vi "TestTCP.vi"() -> ()   [LabVIEW 2020]
panel:
  out "error out":errorcluster
  out "data out1":string
  out "loop2":i32
  out "loop1":i32
  out "data out 2":string
  in  "Stop loop 2":bool
  in  "Stop loop1":bool
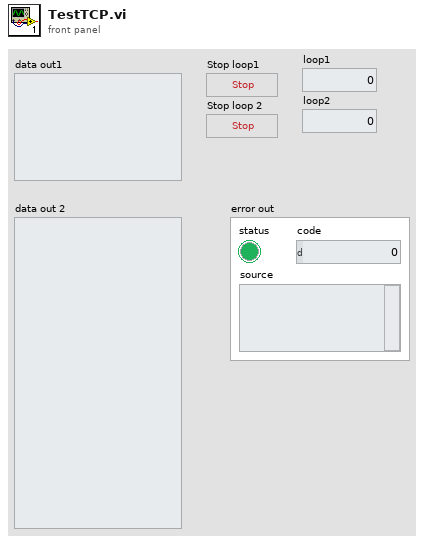
[diagram p1: front panel]
types:
  T1 = enum16{"Standard", "Buffered", "CRLF", "Immediate"}
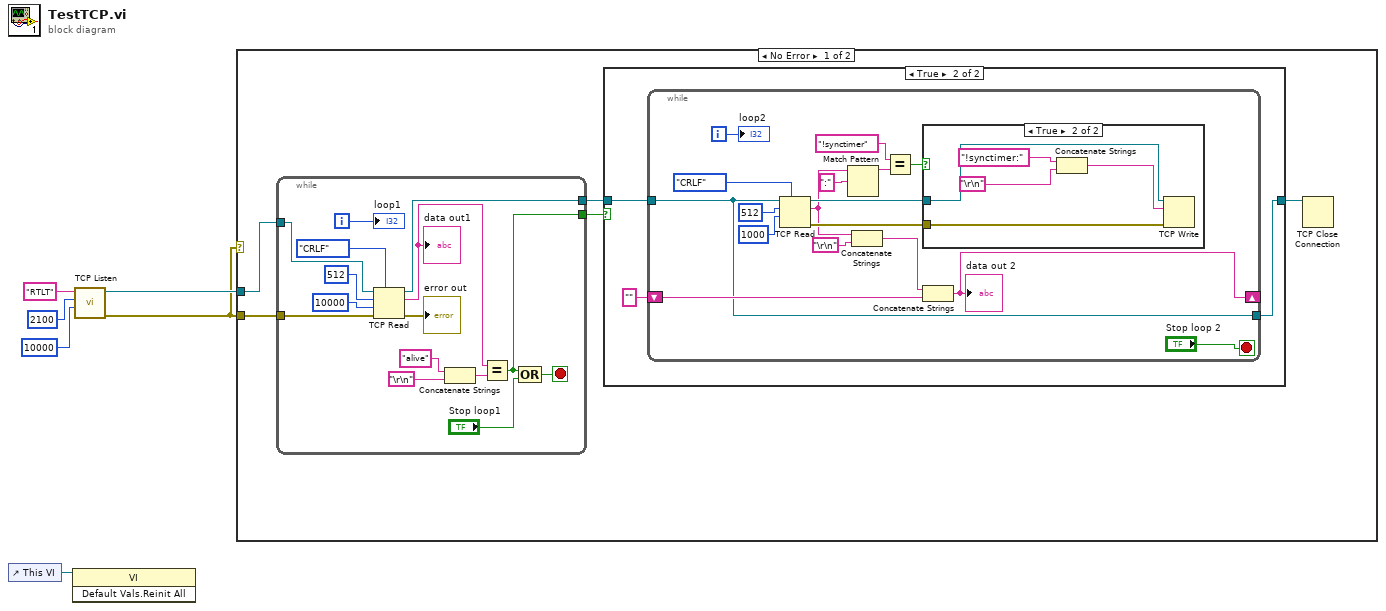
[diagram p0: block diagram]
diagram:
  n1 = control-ref of="This VI"() -> (w2:refnum<vi>)
  n2 = invoke class="VI" method="Default Vals.Reinit All"(reference=w2) -> ()  [unwired: 2 in, 3 out]
  n3 = call <vilib>:"TCP Listen.vi"("timeout ms (wait forever: -1)"=10000, "port"=u16 2100, "service name"="RTLT") -> ("error out"=w1:errorcluster, "connection ID"=w3:refnum<k5>)  [unwired: 4 in, 3 out]
  n4 = case shown="No Error" w1 {
    tunnel: w3 -> [w11 _]
    tunnel: w1 -> [w10 _]
    frame No Error {
      n5 = while {
        tunnel: w11 -> [w52]
        tunnel: w10 -> [w51]
        tunnel: [w42] -> w9
        tunnel: [w40] -> w8
        i -> [w39]
        stop <- w41 stop-if-true
        n6 = TCP Read(connection ID=w52, bytes to read=512, error in (no error)=w51, 7:T1."CRLF" ("mode (standard)"), 9:10000 ("timeout ms (25000)")) -> (connection ID out=w40:refnum<k5>, data out=w48:string, error out=→"error out":errorcluster)
        "data out1" <- w48
        n7 = Concatenate Strings("alive" ("string"), "\r\n") -> (w45:string)
        n8 = Equal?(x=w48, y=w45) -> (x = y?=w42:bool)
        n9 = Compound Arithmetic op=OR(w42, "Stop loop1") -> (w41:bool)
        "loop1" <- w39
      }
      n10 = case shown="True" w9 {
        tunnel: w8 -> [w12 w15]
        tunnel: [w12 w13] -> w7
        frame False {
        }
        frame True {
          n11 = while {
            tunnel: w15 -> [w20]
            shift-right: [w21] -> _
            shift-left: "" ("data out") -> [w22]
            tunnel: [w20] -> w13
            i -> [w25]
            stop <- "Stop loop 2" stop-if-true
            n12 = TCP Read(connection ID=w20, bytes to read=512, 7:T1."CRLF" ("mode (standard)"), 9:1000 ("timeout ms (25000)")) -> (connection ID out=w27:refnum<k5>, data out=w19:string, error out=w26:errorcluster)  [unwired: 1 in]
            n13 = Match Pattern(string=w19, regular expression=":") -> (before substring=w17:string)  [unwired: 1 in, 3 out]
            n14 = Concatenate Strings(w19, "\r\n") -> (w23:string)
            n15 = Equal?(x="!synctimer", y=w17) -> (x = y?=w28:bool)
            n16 = case shown="True" w28 {
              tunnel: w27 -> [_ w37]
              tunnel: w26 -> [_ w33]
              frame False {
              }
              frame True {
                n17 = Concatenate Strings("!synctimer:" ("data in"), "\r\n") -> (w34:string)
                n18 = TCP Write(connection ID=w37, data in=w34, error in (no error)=w33) -> ()  [unwired: 1 in, 3 out]
              }
            }
            n19 = Concatenate Strings(w23, w22) -> (w21:string)
            "data out 2" <- w21
            "loop2" <- w25
          }
        }
      }
      n20 = TCP Close Connection(connection ID=w7) -> ()  [unwired: 2 in, 2 out]
    }
    frame Error {
    }
  }
